vi "Tile.vi"(0 "LV MDI.lvclass":refnum<class "LV MDI.lvclass">, 5 "Tile Direction":u16(ring) items=["Horizontal", "Vertical"], 11 "error in (no error)":errorcluster) -> (4 "LV MDI.lvclass":refnum<class "LV MDI.lvclass">, 15 "error out":errorcluster)   [LabVIEW 2016, in "LV MDI.lvclass"]
uses:
  LV MDI.lvclass
  LV MDI.lvclass/LV MDI.ctl
  user32.dll
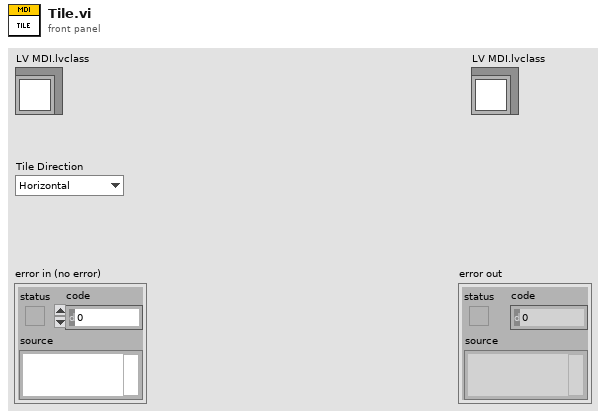
[diagram p1: front panel]
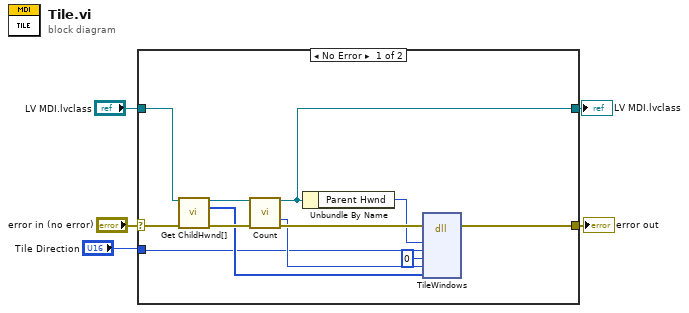
[diagram p0: block diagram]
diagram:
  n1 = case shown="No Error" "error in (no error)" {
    selector: "error in (no error)" -> [w17 w19]
    tunnel: [w10 w19] -> w4
    tunnel: [w13 w18] -> w2
    tunnel: "LV MDI.lvclass" -> [w15 w18]
    tunnel: "Tile Direction" -> [w6 _]
    frame No Error {
      n2 = call "Get ChildHwnd[].vi"("LV MDI in"=w15, "error in (no error)"=w17) -> ("LV MDI out"=w14:refnum<class "LV MDI.lvclass">, "ChildHwnd[]"=w12:u32[], "error out"=w16:errorcluster)  [unwired: 11 in]
      n3 = call "Count.vi"("LV MDI in"=w14, "error in (no error)"=w16) -> ("LV MDI out"=w13:refnum<class "LV MDI.lvclass">, "Count"=w9:i32, "error out"=w11:errorcluster)  [unwired: 11 in]
      n4 = Unbundle By Name(w13) -> ("Parent Hwnd"=w7:i32)
      n5 = dll-call lib="user32.dll" fn="TileWindows"(error in=w11, "hwndParent"=w7, "wHow"=w6, "lpRect"=0 ("wHow"), "cKids"=w9, "lpKids"=w12) -> (error out=w10:errorcluster)  [unwired: 8 in, 1 out]
    }
    frame Error {
    }
  }
  "error out" <- w4
  "LV MDI.lvclass" <- w2
